vi "cell pair to sonde value cluster.vi"(6 "Initial Value":dbl, 7 "Cluster in":T1 {"%" format="%_2f%%"; "Value" format="%_4g"}, 8 "error in":errorcluster, 9 "start index":i32=6, 10 "Array":string[](array[string]), 11 "tolerance limit":dbl) -> (0 "error out":errorcluster, 1 "Tolerance":bool, 2 "%":dbl, 3 "Value":dbl, 5 "Cluster Out":T1 {"%" format="%_2f%%"; "Value" format="%_4g"})   [LabVIEW 2016]
uses:
  Sonde Value Percent Tol.ctl
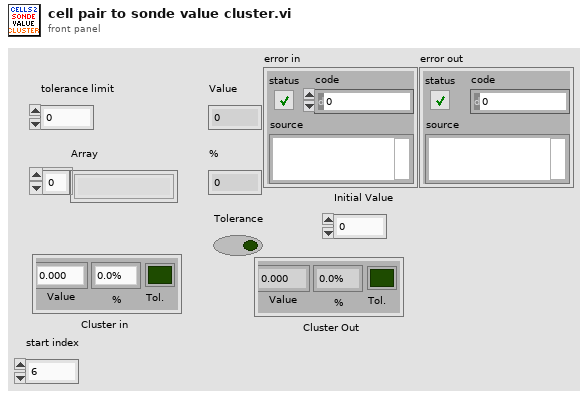
[diagram p1: front panel]
types:
  T1 = typedef "Sonde Value Percent Tol.ctl" = cluster{"Value":dbl, "%":dbl, "Tol.":bool}
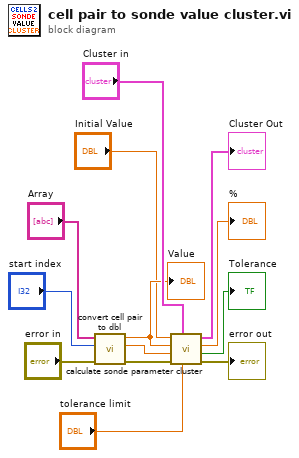
[diagram p0: block diagram]
diagram:
  n1 = call "convert cell pair to dbl.vi"("error in"="error in", "start index"="start index", "Array"="Array") -> ("error out"=w9:errorcluster, "Numeric of start index +1"=w5:dbl, "Numeric of start index"=w7:dbl)  [unwired: 6 in]
  "Value" <- w7
  n2 = call "calculate sonde parameter cluster.vi"("tolerance limit"="tolerance limit", "Cluster in"="Cluster in", "error in (no error)"=w9, "Read % value"=w5, "Read Value"=w7, "Initial Value"="Initial Value") -> ("error out"=→"error out":errorcluster, "Tolerance"=→"Tolerance":bool, "%"=→"%":dbl, "Cluster Out"=→"Cluster Out":T1)  [unwired: 2 in]
